vi "PH_Beckhoff.scale analog Values.vi"(3 "DIM value":dbl, 4 "Beckhoff value":u32, 5 "Sca Type":T1) -> (0 "Scaled Beckhoff value":u32, 1 "Scaled DIM value":dbl, 2 "Scaling":string)   [LabVIEW 2014, in "PH_Beckhoff.lvlib"]
doc: "This VI relates the scaling to the scaling type."
uses:
  PH_Beckhoff.lvlib
  PH_Beckhoff.Scaling Type.ctl
  instr.lib/Beckhoff/Beckhoff - Driver np.lvlib
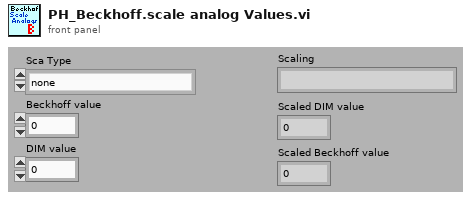
[diagram p1: front panel]
types:
  T1 = typedef "PH_Beckhoff.lvlib/PH_Beckhoff.Scaling Type.ctl" = enum16{"none", "0 ... 15 Bit -> 0 ... 5", "0 ... 15 Bit -> 0 ... 10", "0 ... 15 Bit -> 0 ... 25", "0 ... 15 Bit -> 4 ... 20", "0 ... 15 Bit -> 0 ... 1", "0 ... 15 Bit -> 0 ... 20000", "0 ... 15 Bit -> 0 ... 24000"}
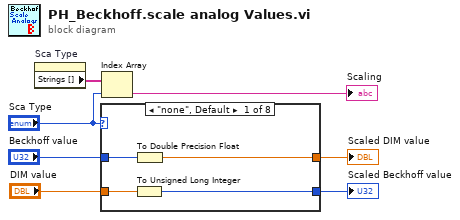
[diagram p0: block diagram]
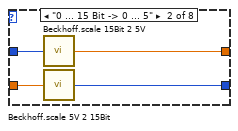
[diagram p2: hidden frame]
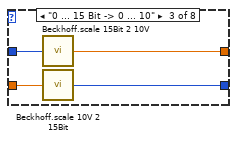
[diagram p3: hidden frame]
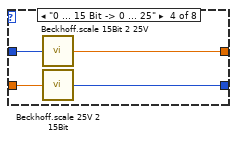
[diagram p4: hidden frame]
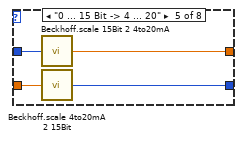
[diagram p5: hidden frame]
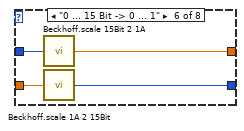
[diagram p6: hidden frame]
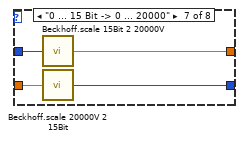
[diagram p7: hidden frame]
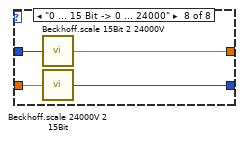
[diagram p8: hidden frame]
diagram:
  n1 = property on="Sca Type" class="Enum (strict)"() -> ("Strings []"=w3:string[])  [unwired: 2 in, 2 out]
  n2 = case shown="\"none\", Default" "Sca Type" {
    tunnel: "Beckhoff value" -> [w11 w15 w19 w23 w27 w31 w35 w39]
    tunnel: [w10 w14 w18 w22 w26 w30 w34 w38] -> w4
    tunnel: "DIM value" -> [w9 w13 w17 w21 w25 w29 w33 w37]
    tunnel: [w8 w12 w16 w20 w24 w28 w32 w36] -> w7
    frame "none", Default {
      n3 = To Unsigned Long Integer(number=w9) -> (unsigned 32bit integer=w8:u32)
      n4 = To Double Precision Float(number=w11) -> (double precision float=w10:dbl)
    }
    frame "0 ... 15 Bit -> 0 ... 5" {
      n5 = call "Beckhoff.scale 15Bit 2 5V.vi"("15Bit Value"=w15) -> ("Scaled Value [V]"=w14:dbl)
      n6 = call "Beckhoff.scale 5V 2 15Bit.vi"("Voltage [V]"=w13) -> ("15 Bit Value"=w12:u32)
    }
    frame "0 ... 15 Bit -> 0 ... 10" {
      n7 = call "Beckhoff.scale 15Bit 2 10V.vi"("15Bit Value"=w19) -> ("Scaled Value [V]"=w18:dbl)
      n8 = call "Beckhoff.scale 10V 2 15Bit.vi"("Voltage [V]"=w17) -> ("15 Bit Value"=w16:u32)
    }
    frame "0 ... 15 Bit -> 0 ... 25" {
      n9 = call "Beckhoff.scale 15Bit 2 25V.vi"("15Bit Value"=w23) -> ("Scaled Value [V]"=w22:dbl)
      n10 = call "Beckhoff.scale 25V 2 15Bit.vi"("Voltage [V]"=w21) -> ("15 Bit Value"=w20:u32)
    }
    frame "0 ... 15 Bit -> 4 ... 20" {
      n11 = call "Beckhoff.scale 15Bit 2 4to20mA.vi"("15Bit Value"=w27) -> ("Scaled Value [mA]"=w26:dbl)
      n12 = call "Beckhoff.scale 4to20mA 2 15Bit.vi"("Current [mA]"=w25) -> ("15 Bit Value"=w24:u32)
    }
    frame "0 ... 15 Bit -> 0 ... 1" {
      n13 = call "Beckhoff.scale 15Bit 2 1A.vi"("15Bit Value"=w31) -> ("Scaled Value [A]"=w30:dbl)
      n14 = call "Beckhoff.scale 1A 2 15Bit.vi"("Current [A]"=w29) -> ("15 Bit Value"=w28:u32)
    }
    frame "0 ... 15 Bit -> 0 ... 20000" {
      n15 = call "Beckhoff.scale 15Bit 2 20000V.vi"("15Bit Value"=w35) -> ("Scaled Value [V]"=w34:dbl)
      n16 = call "Beckhoff.scale 20000V 2 15Bit.vi"("Voltage [V]"=w33) -> ("15 Bit Value"=w32:u32)
    }
    frame "0 ... 15 Bit -> 0 ... 24000" {
      n17 = call "Beckhoff.scale 15Bit 2 24000V.vi"("15Bit Value"=w39) -> ("Scaled Value [V]"=w38:dbl)
      n18 = call "Beckhoff.scale 24000V 2 15Bit.vi"("Voltage [V]"=w37) -> ("15 Bit Value"=w36:u32)
    }
  }
  "Scaled Beckhoff value" <- w7
  "Scaled DIM value" <- w4
  n19 = Index Array(array=w3, index="Sca Type") -> (element=→"Scaling":string)
